vi "pump calibration dialog.vi"() -> ()   [LabVIEW 2012]
uses:
  calibration commands.ctl
  calibration values.ctl
panel:
  in  "Calculate RPM Calibration":bool
  in  "RPM Calibration":T1
  in  "STAMP Calibration":bool
  in  "STAMP intercept":dbl
  in  "STAMP slope":dbl=1.0
  in  "OK Button":bool
  in  "Set to Default":bool
  in  "Flow Calibration":T2
  in  "Save Calibration":bool
  # "scaled 0-100"
  # "scaled 0-100"
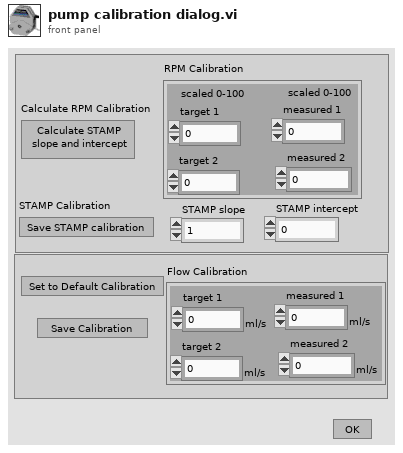
[diagram p1: front panel]
types:
  T1 = cluster{"target 1":dbl, "target 2":dbl, "measured 1":dbl, "measured 2":dbl}
  T2 = typedef "calibration values.ctl" = cluster{"target 1":dbl[unit], "target 2":dbl[unit], "measured 1":dbl[unit], "measured 2":dbl[unit]}
  T3 = typedef "calibration commands.ctl" = enum16{"Get ini Path", "Save default values", "Save new calibration", "Read calibration", "Apply calibration", "Read STAMP mb", "Write STAMP mb"}
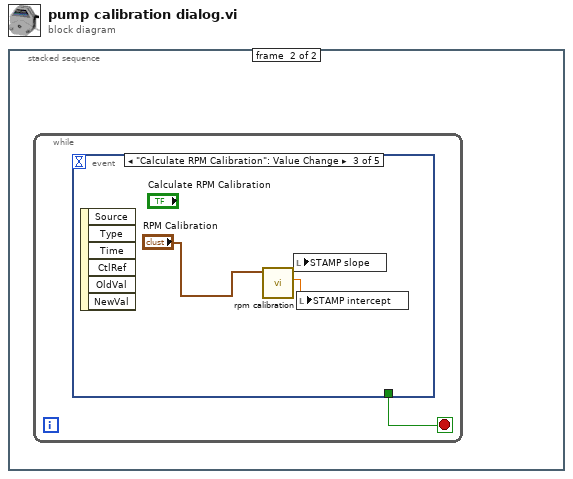
[diagram p0: block diagram]
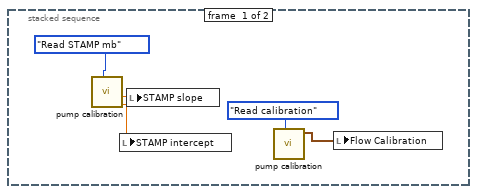
[diagram p2: hidden frame]
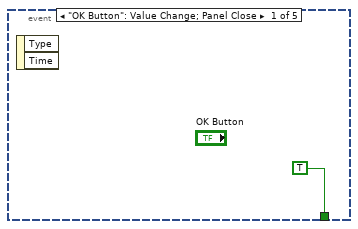
[diagram p3: hidden frame]
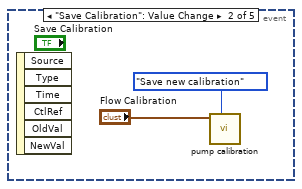
[diagram p4: hidden frame]
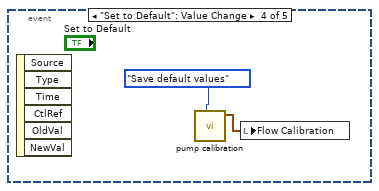
[diagram p5: hidden frame]
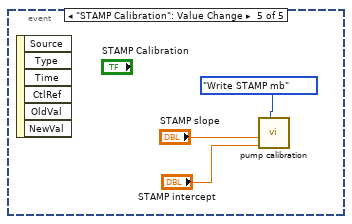
[diagram p6: hidden frame]
diagram:
  n1 = stacked-sequence {
    frame #0 {
      n2 = call "pump calibration.vi"("pump cal command"=calibration_commands."Read STAMP mb") -> ("STAMP intercept out"=w3:dbl, "STAMP slope out"=w2:dbl)  [unwired: 4 in, 2 out]
      n3 = local write "STAMP intercept"(w3) -> ()
      n4 = local write "STAMP slope"(w2) -> ()
      n5 = call "pump calibration.vi"("pump cal command"=calibration_commands."Read calibration") -> ("Pump Calibration out"=w4:T2)  [unwired: 4 in, 3 out]
      n6 = local write "Flow Calibration"(w4) -> ()
    }
    frame #1 {
      n7 = while {
        stop <- w6 stop-if-true
        n8 = event shown="[2] \"Calculate RPM Calibration\": Value Change" {
          selector: _ -> [_ _ _ _ _]
          dyn-events: _ -> [_ _ _ _ _]
          timeout: _ -> [_ _ _ _ _]
          tunnel: [TRUE _ _ _ _] -> w6
          event "OK Button": Value Change; Panel Close {
            n9 = event-data() -> ()  [unwired: 1 in, 2 out]
          }
          event "Save Calibration": Value Change {
            n10 = event-data() -> ()  [unwired: 1 in, 6 out]
            n11 = call "pump calibration.vi"("pump cal command"=calibration_commands."Save new calibration", "Pump Calibration in"="Flow Calibration") -> ()  [unwired: 3 in, 4 out]
          }
          event "Calculate RPM Calibration": Value Change {
            n12 = event-data() -> ()  [unwired: 1 in, 6 out]
            n13 = call "rpm calibration.vi"("RPM Calibration"="RPM Calibration") -> ("STAMP intercept"=w10:dbl, "STAMP slope"=w11:dbl)  [unwired: 9 in]
            n14 = local write "STAMP slope"(w11) -> ()
            n15 = local write "STAMP intercept"(w10) -> ()
          }
          event "Set to Default": Value Change {
            n16 = event-data() -> ()  [unwired: 1 in, 6 out]
            n17 = call "pump calibration.vi"("pump cal command"=calibration_commands."Save default values") -> ("Pump Calibration out"=w13:T2)  [unwired: 4 in, 3 out]
            n18 = local write "Flow Calibration"(w13) -> ()
          }
          event "STAMP Calibration": Value Change {
            n19 = event-data() -> ()  [unwired: 1 in, 6 out]
            n20 = call "pump calibration.vi"("pump cal command"=calibration_commands."Write STAMP mb", "STAMP intercept"="STAMP intercept", "STAMP slope"="STAMP slope") -> ()  [unwired: 2 in, 4 out]
          }
        }
      }
    }
  }
